vi "FgenInstrument_CallInitializeMeasurementLinkSessionWithCreateBehavior_RemoteSessionCreated.vi"(8 "error in":errorcluster) -> (0 "error out":errorcluster, 2 "result":string, 3 "pass":bool)   [LabVIEW 2020, in "MeasurementServerTests.lvlib"]
uses:
  MeasurementServerTests.lvlib
  Runtime/MeasurementLink Instrument/IInstrument/Initialize Session Behavior.ctl
  Runtime/MeasurementLink niFGEN/Instrument/Instrument.lvclass
  Runtime/MeasurementLink Instrument/IInstrument/IInstrument.lvclass
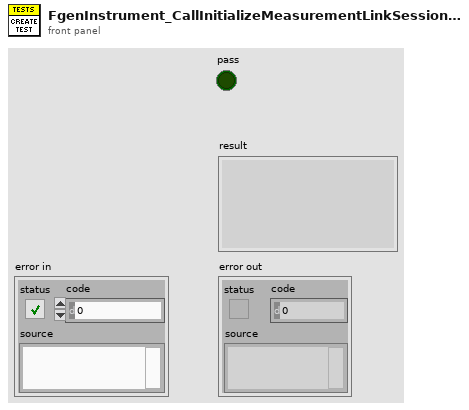
[diagram p1: front panel]
types:
  T1 = typedef "MeasurementLink Instrument.lvlib/IInstrument.lvclass/Remote Connection Options.ctl" = cluster{"session name":string, "address":string, "port":u32}
  T2 = typedef "MeasurementLink Instrument.lvlib/IInstrument.lvclass/Initialize Session Behavior.ctl" = enum16{"Create Session", "Attach Session"}
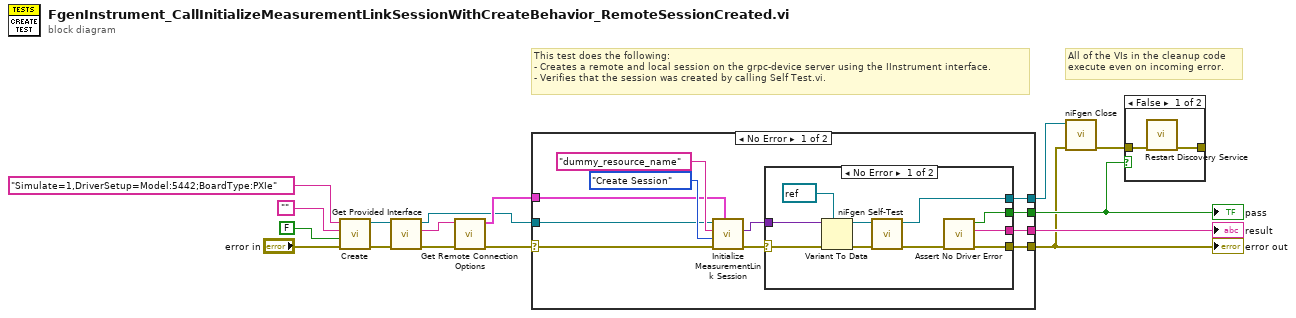
[diagram p0: block diagram]
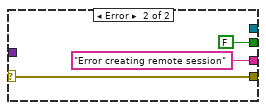
[diagram p2: hidden frame]
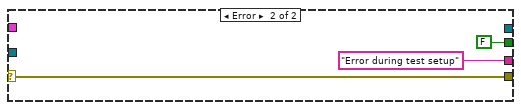
[diagram p3: hidden frame]
diagram:
  # "All of the VIs in the cleanup code\nexecute even on incoming error."
  # "This test does the following:\n- Creates a remote and local session on the grpc-device server using the IInstrument interface.\n- Verifies that the session was created by calling Self Test.vi."
  n1 = call "Create.vi"("error in"="error in", "reset"=FALSE, "channel name"="", "option string"="Simulate=1,DriverSetup=Model:5442;BoardType:PXIe") -> ("error out"=w6:errorcluster, "instrument out"=w5:refnum<class "Instrument.lvclass">)  [unwired: 6 in]
  n2 = call-dynamic "Get Provided Interface.vi"("error in"=w6, "instrument in"=w5) -> ("error out"=w14:errorcluster, "provided interface"=w15:string, "instrument out"=w11:refnum<class "Instrument.lvclass">)  [unwired: 7 in]
  n3 = call "Get Remote Connection Options.vi"("error in"=w14, "provided interface"=w15) -> ("error out"=w13:errorcluster, "remote connection options"=w12:T1)  [unwired: 8 in]
  n4 = case shown="No Error" w13 {
    selector: w13 -> [w20 w41]
    tunnel: [w26 w41] -> w8
    tunnel: [w27 FALSE] -> w9
    tunnel: [w25 "Error during test setup" ("f")] -> w16
    tunnel: w12 -> [w19 _]
    tunnel: w11 -> [w18 _]
    tunnel: [w17 _] -> w1
    frame No Error {
      n5 = call-dynamic "Initialize MeasurementLink Session.vi"("remote connection options"=w19, "error in"=w20, "initialize session behavior"=Initialize_Session_Behavior."Create Session", "resource name"="dummy_resource_name", "instrument in"=w18) -> ("error out"=w23:errorcluster, "session out"=w24:variant)  [unwired: 4 in, 1 out]
      n6 = case shown="No Error" w23 {
        selector: w23 -> [w36 w39]
        tunnel: [w28 FALSE] -> w27
        tunnel: [w30 w39] -> w26
        tunnel: [w29 "Error creating remote session"] -> w25
        tunnel: w24 -> [w37 _]
        tunnel: [w32 _] -> w17
        frame No Error {
          n7 = Variant To Data(error in=w36, type=refnum<k15> refnum ("Instrument Handle Out"), Variant=w37) -> (data=w34:refnum<k15>, error out=w35:errorcluster)
          n8 = call <instrlib>:"niFgen Self-Test.vi"("error in (no error)"=w35, "Instrument Handle"=w34) -> ("error out"=w31:errorcluster, "Instrument Handle Out"=w32:refnum<k15>)  [unwired: 6 in, 2 out]
          n9 = call "Assert No Driver Error.vi"("error in"=w31) -> ("error out"=w30:errorcluster, "result"=w29:string, "pass?"=w28:bool)  [unwired: 8 in]
        }
        frame Error {
        }
      }
    }
    frame Error {
    }
  }
  "error out" <- w8
  "pass" <- w9
  "result" <- w16
  n10 = call <instrlib>:"niFgen Close.vi"("error in (no error)"=w8, "Instrument Handle"=w1) -> ("error out"=w10:errorcluster)  [unwired: 9 in]
  n11 = case shown="False" w9 {
    tunnel: w10 -> [w45 _]
    tunnel: [w44 _] -> _
    frame False {
      n12 = call "Restart Discovery Service.vi"("error in"=w45) -> ("error out"=w44:errorcluster)  [unwired: 10 in]
    }
    frame True {
    }
  }
